vi "DHE_IRExpose.vi"(2 "error in":errorcluster, 4 "fd":i32) -> (0 "error out":errorcluster)   [LabVIEW 2016]
uses:
  DBSHAND/private/vis/DatabaseHand_Element_Set(I32).vi
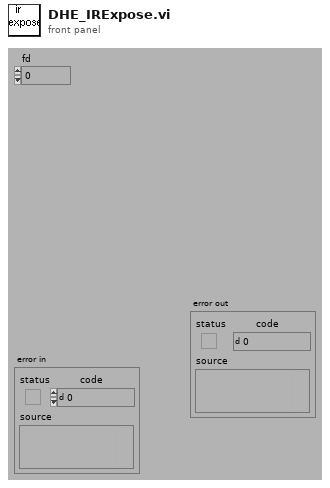
[diagram p1: front panel]
types:
  T1 = typedef "DatabaseHand_RefNum.ctl" = refnum<vi>
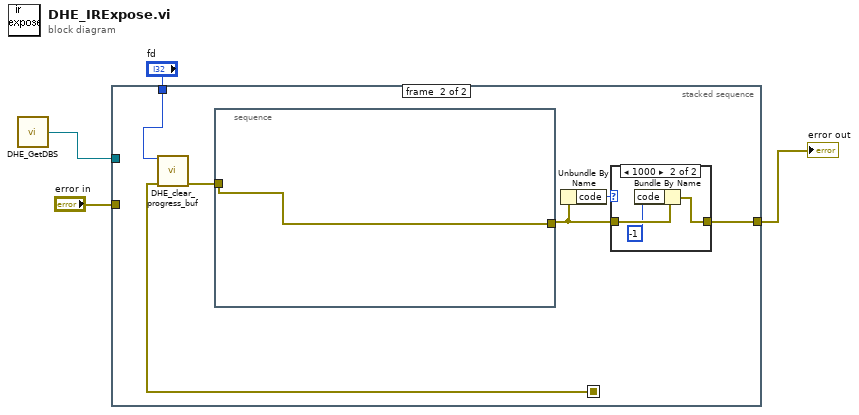
[diagram p0: block diagram]
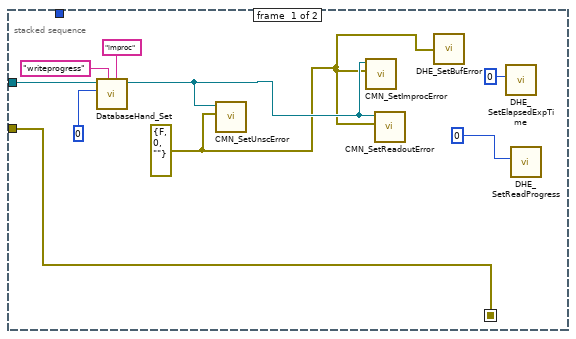
[diagram p2: hidden frame]
diagram:
  n1 = call "DHE_GetDBS.vi"() -> ("DHE_DBSRef"=w1:T1)  [unwired: 9 out]
  n2 = stacked-sequence {
    seq-local: [w13 _] -> [_ w14]
    tunnel: "error in" -> [w13 _]
    tunnel: "fd" -> [_ w16]
    tunnel: [_ w19] -> w2
    tunnel: w1 -> [w10 _]
    frame #0 {
      w6 = errorcluster {"status"=FALSE, "code"=0, "source"=""} ("readout Error")
      n3 = call-poly "DatabaseHand_Set.vi"("group"="improc", "name"="writeprogress" ("value"), "value"=0, "Database RefNum in"=w10) -> ("Database RefNum out"=w8:T1)  [unwired: 4 in, 3 out]
      n4 = call "CMN_SetUnscError.vi"("unsc error"=w6, "Database RefNum in"=w8) -> ()  [unwired: 1 in, 9 out]
      n5 = call "CMN_SetImprocError.vi"("improc error"=w6, "Database RefNum in"=w8) -> ()  [unwired: 1 in, 9 out]
      n6 = call "CMN_SetReadoutError.vi"("readout error"=w6, "Database RefNum in"=w8) -> ()  [unwired: 1 in, 9 out]
      n7 = call "DHE_SetBufError.vi"("DHE_BufError"=w6) -> ()  [unwired: 9 out]
      n8 = call "DHE_SetElapsedExpTime.vi"("ElapsedExpTime"=u32 0 ("ElapsedExp")) -> ()  [unwired: 11 out]
      n9 = call "DHE_SetReadProgress.vi"("ReadProgress"=u8 0 ("Readprogress")) -> ()  [unwired: 11 out]
    }
    frame #1 {
      n10 = call "DHE_clear_progress_buf.vi"("fd"=w16, "error in (no error)"=w14) -> ("error out"=w15:errorcluster)  [unwired: 13 out]
      n11 = stacked-sequence {
        tunnel: w15 -> [w24]
        tunnel: [w24] -> w18
        frame #0 {
        }
      }
      n12 = Unbundle By Name(w18) -> ("code"=w17:i32)
      n13 = case shown="1000" w17 {
        tunnel: w18 -> [w20 w23]
        tunnel: [w20 w22] -> w19
        frame Default {
        }
        frame 1000 {
          n14 = Bundle By Name(cluster=w23, "code"=-1) -> (w22:errorcluster)
        }
      }
    }
  }
  "error out" <- w2
